vi "DMM Continuous Read.vi"() -> ()   [LabVIEW 2010]
panel:
  out "Fringe Size (Vpp)":dbl
  in  "stop":bool
  out "Waveform Chart":dbl(graph)
  in  "milliseconds to wait":u32=20
  out "# of points taken":i32
  out "Value":dbl
  out "Reading (string)":string
  out "substring (Units)":string
  out "error out":errorcluster
  out "read buffer":string
  out "return count":u32
  in  "byte count":u32=5000000
  in  "VISA resource name":refnum<visa-resource-name>="GPIB0::25::INSTR"
  in  "write buffer":string="G0"
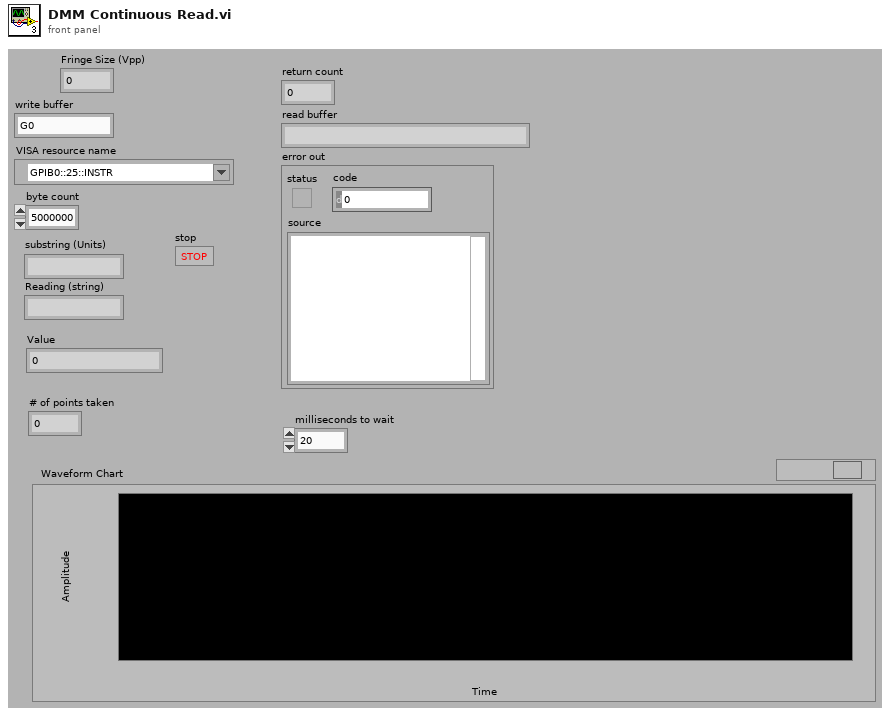
[diagram p1: front panel]
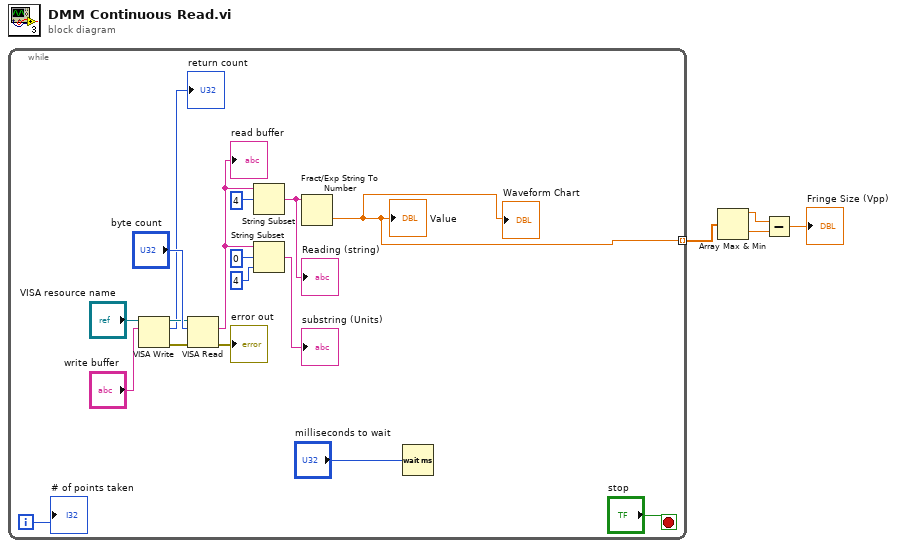
[diagram p0: block diagram]
diagram:
  n1 = while {
    tunnel: [w5] -> w4 mode=indexing
    i -> [w8]
    stop <- "stop" stop-if-true
    n2 = VISA Write(VISA resource name="VISA resource name", write buffer="write buffer") -> (VISA resource name out=w18:refnum<visa-resource-name>, return count=→"return count":u32, error out=w16:errorcluster)  [unwired: 1 in]
    n3 = VISA Read(VISA resource name=w18, byte count="byte count", error in (no error)=w16) -> (read buffer=w11:string, error out=→"error out":errorcluster)  [unwired: 2 out]
    "read buffer" <- w11
    n4 = String Subset(string=w11, offset (0)=4) -> (substring=w9:string)  [unwired: 1 in]
    "Reading (string)" <- w9
    n5 = String Subset(string=w11, offset (0)=0, length (rest)=4 ("length (rest)")) -> (substring=→"substring (Units)":string)
    n6 = Fract/Exp String To Number(string=w9) -> (number=w5:dbl)  [unwired: 3 in, 1 out]
    "Value" <- w5
    "Waveform Chart" <- w5
    n7 = Wait (ms)(milliseconds to wait="milliseconds to wait") -> ()  [unwired: 1 out]
    "# of points taken" <- w8
  }
  n8 = Array Max & Min(array=w4) -> (max value=w3:dbl, min value=w2:dbl)  [unwired: 2 out]
  n9 = Subtract(x=w3, y=w2) -> (x-y=→"Fringe Size (Vpp)":dbl)
